vi "Test Triangle Class.vi"(8 "error in (no error)":errorcluster, 11 "TestCase in":refnum<class "Test FGEN.lvclass">) -> (0 "error out":errorcluster, 3 "TestCase out":refnum<class "Test FGEN.lvclass">)   [LabVIEW 2020, in "Test FGEN.lvclass"]
uses:
  Test FGEN.lvclass
  Libraries/FGen/Generador/Generador.lvclass
  <vilib>/addons/_JKI Toolkits/VI Tester/TestCase.llb/TestCase.lvclass
  C:/Program Files (x86)/National Instruments/LabVIEW 2020/vi.lib/addons/_JKI Toolkits/VI Tester/TestCase.llb/TestCase.lvclass
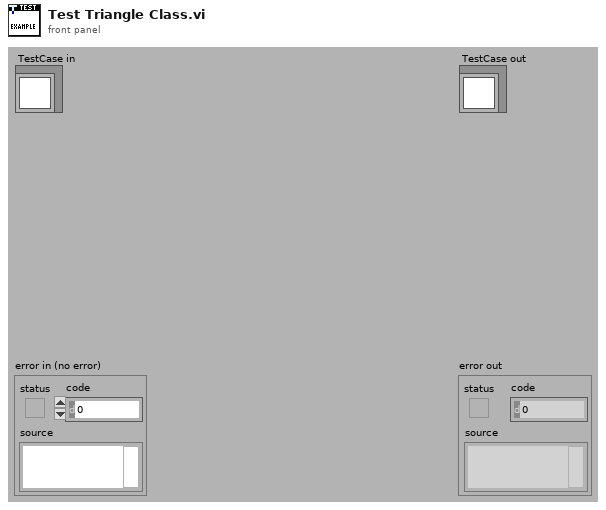
[diagram p1: front panel]
types:
  T1 = enum16{"Sine Wave", "Triangle Wave", "Square Wave", "Sawtooth Wave"}
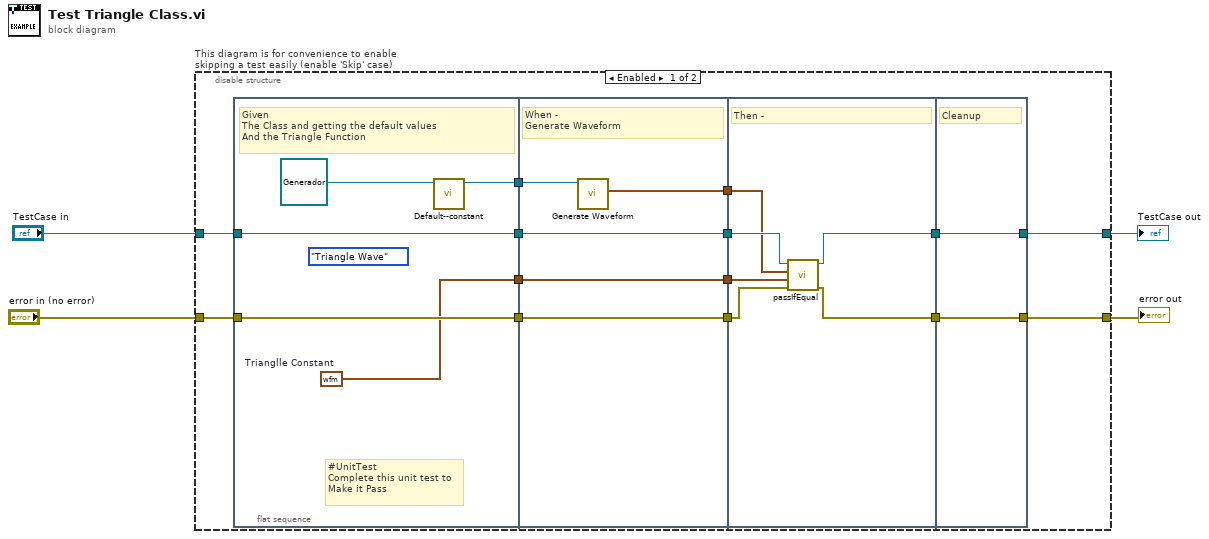
[diagram p0: block diagram]
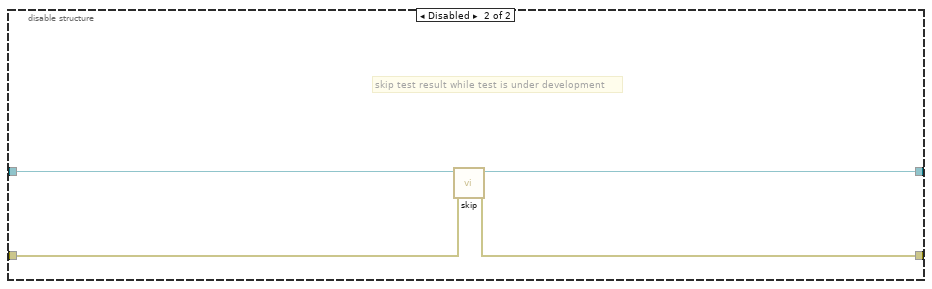
[diagram p2: hidden frame]
diagram:
  n1 = disable-structure "This diagram is for convenience to enable skipping a test easily (enable 'Skip' case)" shown="Enabled" {
    disable-tunnel: "TestCase in" -> [w14 w40]
    disable-tunnel: [w12 w38] -> w1
    disable-tunnel: [w13 w39] -> w3
    disable-tunnel: "error in (no error)" -> [w11 w37]
    frame Enabled {
      n2 = flat-sequence {
        tunnel: w14 -> [w23]
        tunnel: [w23] -> w18
        tunnel: w11 -> [w22]
        tunnel: [w22] -> w9
        tunnel: [w21] -> w7
        tunnel: [w20] -> w6
        tunnel: [w28] -> w17
        tunnel: w18 -> [w28]
        tunnel: [w27] -> w10
        tunnel: w9 -> [w27]
        tunnel: [w26] -> w8
        tunnel: w7 -> [w26]
        tunnel: w6 -> [w25]
        tunnel: [w24] -> w5
        tunnel: [w33] -> w16
        tunnel: [w32] -> w15
        tunnel: w17 -> [w34]
        tunnel: w10 -> [w31]
        tunnel: w8 -> [w29]
        tunnel: w5 -> [w30]
        tunnel: [w35] -> w13
        tunnel: [w36] -> w12
        tunnel: w16 -> [w36]
        tunnel: w15 -> [w35]
        frame #0 {
          w21 = waveform(dbl) {"t0"=timestamp(0 s since 1904-01-01), "dt"=1.0, "Y"=[]}  # Trianglle Constant
          (unwired) T1."Triangle Wave" ("signal type")
          # "#UnitTest\nComplete this unit test to\nMake it Pass"
          # "Given\nThe Class and getting the default values\nAnd the Triangle Function"
          n3 = call-dynamic "Default--constant.vi"("Generator in"=refnum<class "Generador.lvclass"> refnum ("FGen.lvlib:Generator")) -> ("Generator out"=w20:refnum<class "Generador.lvclass">)  [unwired: 9 in, 1 out]
        }
        frame #1 {
          # "When -\nGenerate Waveform"
          n4 = call "Generate Waveform.vi"("Generator in"=w25) -> ("Waveform"=w24:waveform(dbl))  [unwired: 8 in, 2 out]
        }
        frame #2 {
          # "Then -"
          n5 = call-dynamic "passIfEqual.vi"("error in (no error)"=w31, "y"=w29, "x"=w30, "TestCase in"=w34) -> ("error out"=w32:errorcluster, "TestCase out"=w33:refnum<class "Test FGEN.lvclass">)  [unwired: 6 in]
        }
        frame #3 {
          # "Cleanup"
        }
      }
    }
    frame Disabled {
      # "skip test result while test is under development"
      n6 = call <vilib>:"skip.vi"("error in (no error)"=w37, "TestCase in"=w40) -> ("error out"=w39:errorcluster, "TestCase out"=w38:refnum<class "Test FGEN.lvclass">)  [unwired: 8 in]
    }
  }
  "error out" <- w3
  "TestCase out" <- w1
